vi "FGV_COMinfo to file.vi"(7 "Enum":enum16{"Open", "Write", "Close"}(ring), 8 "error in (no error)":errorcluster, 10 "Data":string, 11 "Path":path) -> (0 "error out":errorcluster)   [LabVIEW 2017]
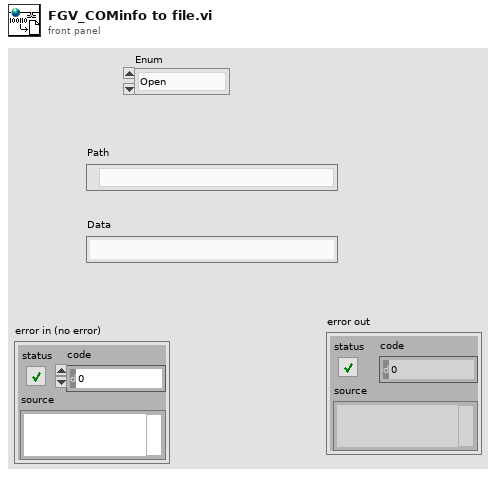
[diagram p1: front panel]
types:
  T1 = enum16{"open", "replace", "create", "open or create", "replace or create", "replace or create with confirmation"}
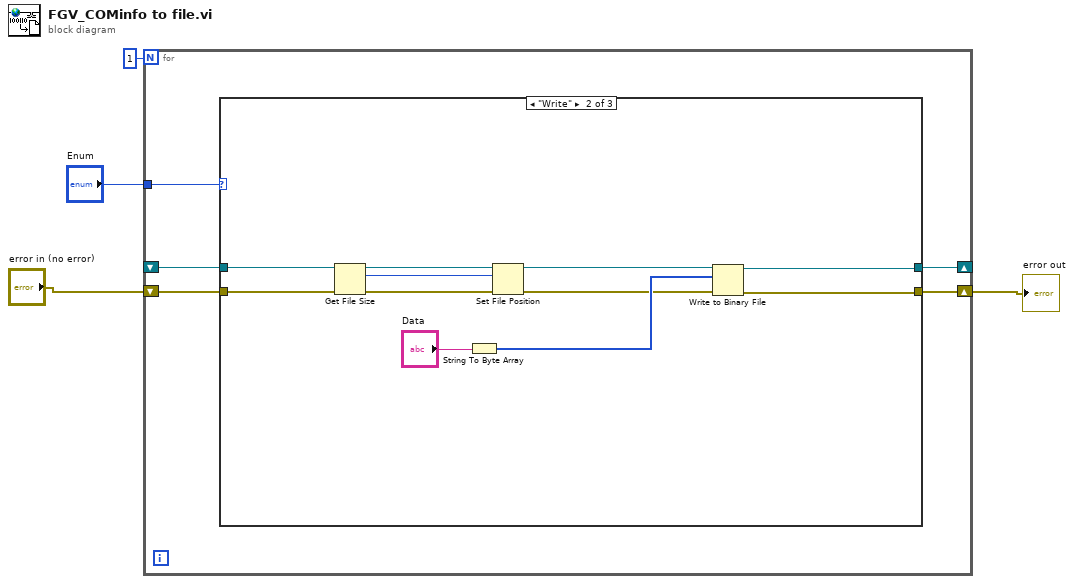
[diagram p0: block diagram]
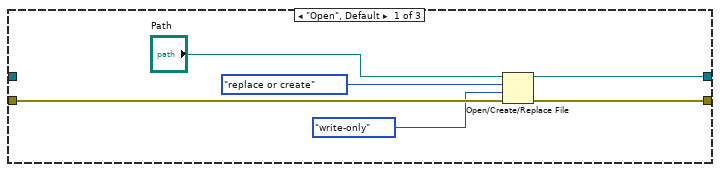
[diagram p2: hidden frame]
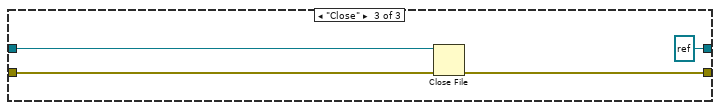
[diagram p3: hidden frame]
diagram:
  n1 = for {
    N: 1 -> [_]
    shift-right: [w9] -> _
    shift-left: _ -> [w8]
    tunnel: "Enum" -> [w7]
    shift-right: [w6] -> w2
    shift-left: "error in (no error)" -> [w5]
    n2 = case shown="\"Write\"" w7 {
      tunnel: [w15 w25 refnum<file> refnum ("refnum out")] -> w9
      tunnel: w8 -> [_ w26 w27]
      tunnel: [w12 w24 w29] -> w6
      tunnel: w5 -> [w11 w18 w30]
      frame "Open", Default {
        n3 = Open/Create/Replace File(file path (use dialog)="Path", error in=w11, operation (0:open)=T1."replace or create", access (0:read/write)=enum16{"read/write", "read-only", "write-only"}."write-only") -> (refnum out=w15:refnum<file>, error out=w12:errorcluster)  [unwired: 2 in, 1 out]
      }
      frame "Write" {
        n4 = Get File Size(file=w26, error in=w18) -> (refnum out=w19:refnum<file>, size (in bytes)=w16:i64, 0:w17:errorcluster)
        n5 = String To Byte Array(string="Data") -> (unsigned byte array=w22:u8[])
        n6 = Set File Position(offset (in bytes) (0)=w16, refnum=w19, error in=w17) -> (refnum out=w21:refnum<file>, error out=w20:errorcluster)  [unwired: 1 in]
        n7 = Write to Binary File(file (use dialog)=w21, data=w22, error in=w20) -> (refnum out=w25:refnum<file>, error out=w24:errorcluster)  [unwired: 3 in, 1 out]
      }
      frame "Close" {
        n8 = Close File(refnum=w27, error in=w30) -> (error out=w29:errorcluster)  [unwired: 1 out]
      }
    }
  }
  "error out" <- w2
